vi "Sensor Specification.vi"(8 "error in (no error)":errorcluster, 11 "VISA resource name":refnum<visa-resource-name>) -> (0 "error out":errorcluster, 2 "Instrument Specifications":T1, 3 "VISA resource name out":refnum<visa-resource-name>)   [LabVIEW 2014, in "Hokuyo URG Series.lvlib"]
doc: "Returns the specifications of the instrument in a cluster data type. The data returned may need to be manipulated using string functions. Refer to the instrument manual for information on the format of the returned data."
uses:
  Hokuyo URG Series.lvlib
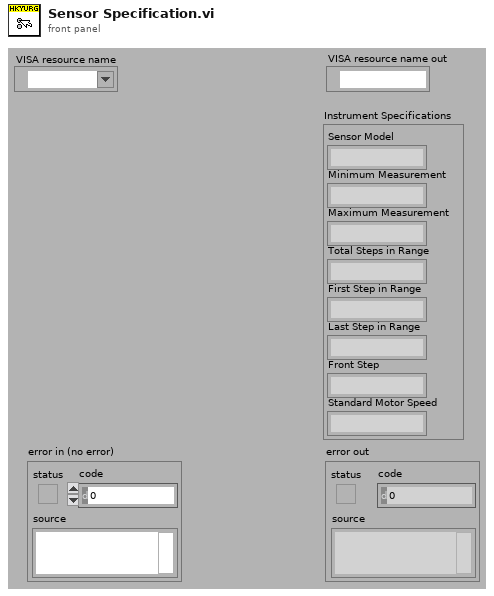
[diagram p1: front panel]
types:
  T1 = cluster{"Sensor Model":string, "Minimum Measurement":string, "Maximum Measurement":string, "Total Steps in Range":string, "First Step in Range":string, "Last Step in Range":string, "Front Step":string, "Standard Motor Speed":string}
  T2 = cluster{"[0]":string, "[1]":string, "[2]":string, "[3]":string, "[4]":string, "[5]":string, "[6]":string, "[7]":string}
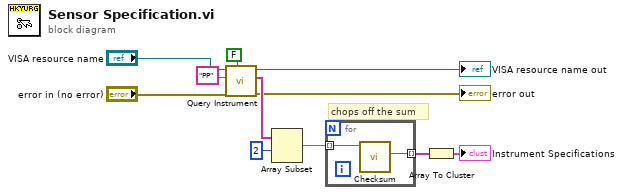
[diagram p0: block diagram]
diagram:
  # "chops off the sum"
  n1 = call "Query Instrument.vi"("Error Query (Enabled)"=FALSE, "error in"="error in (no error)", "Command"="PP", "VISA Resource Name"="VISA resource name") -> ("error out"=→"error out":errorcluster, "Response Strings"=w5:string[], "VISA Resource Name Out"=→"VISA resource name out":refnum<visa-resource-name>)  [unwired: 5 in]
  n2 = Array Subset(array=w5, index=2) -> (w9:string[])  [unwired: 1 in]
  n3 = for {
    tunnel: w9 -> [w13] mode=indexing
    tunnel: [w12] -> w7 mode=indexing
    n4 = call "Checksum.vi"("Input"=w13) -> ("Data Buffer"=w12:string)  [unwired: 9 in, 1 out]
  }
  n5 = Array To Cluster(array=w7) -> (cluster=→"Instrument Specifications":T2)
